vi "Search Or Add Frame.vi"(10 "Detection Frame In 3":T1 {"robots_blue"."height" format="%+4.3f"; "robots_blue"."pixel_y" format="%+4.3f"; "robots_blue"."pixel_x" format="%+4.3f"; "robots_blue"."orientation" format="%+4.3f"; "robots_blue"."y" format="%+4.3f"; "robots_blue"."confidence" format="%4.3f"; "robots_blue"."x" format="%+4.3f"; "robots_yellow"."height" format="%+4.3f"; "robots_yellow"."pixel_y" format="%+4.3f"; "robots_yellow"."pixel_x" format="%+4.3f"; "robots_yellow"."orientation" format="%+4.3f"; "robots_yellow"."y" format="%+4.3f"; "robots_yellow"."confidence" format="%4.3f"; "robots_yellow"."x" format="%+4.3f"}, 11 "Detection Frame In 4":T1[](array[typedef]) {"robots_blue"."height" format="%+4.3f"; "robots_blue"."pixel_y" format="%+4.3f"; "robots_blue"."pixel_x" format="%+4.3f"; "robots_blue"."orientation" format="%+4.3f"; "robots_blue"."y" format="%+4.3f"; "robots_blue"."confidence" format="%4.3f"; "robots_blue"."x" format="%+4.3f"; "robots_yellow"."height" format="%+4.3f"; "robots_yellow"."pixel_y" format="%+4.3f"; "robots_yellow"."pixel_x" format="%+4.3f"; "robots_yellow"."orientation" format="%+4.3f"; "robots_yellow"."y" format="%+4.3f"; "robots_yellow"."confidence" format="%4.3f"; "robots_yellow"."x" format="%+4.3f"}) -> (3 "Detection Frame In 2":T1[](array[typedef]) {"robots_blue"."height" format="%+4.3f"; "robots_blue"."pixel_y" format="%+4.3f"; "robots_blue"."pixel_x" format="%+4.3f"; "robots_blue"."orientation" format="%+4.3f"; "robots_blue"."y" format="%+4.3f"; "robots_blue"."confidence" format="%4.3f"; "robots_blue"."x" format="%+4.3f"; "robots_yellow"."height" format="%+4.3f"; "robots_yellow"."pixel_y" format="%+4.3f"; "robots_yellow"."pixel_x" format="%+4.3f"; "robots_yellow"."orientation" format="%+4.3f"; "robots_yellow"."y" format="%+4.3f"; "robots_yellow"."confidence" format="%4.3f"; "robots_yellow"."x" format="%+4.3f"})   [LabVIEW 2017]
uses:
  SSL Detection Robot.ctl
  SSL Detection Ball.ctl
  SSL Detection Frame.ctl
  <vilib>/Analysis/Matrix/Datatypes/RealMatrix.ctl
  <vilib>/Analysis/Matrix/NI_Matrix.lvlib
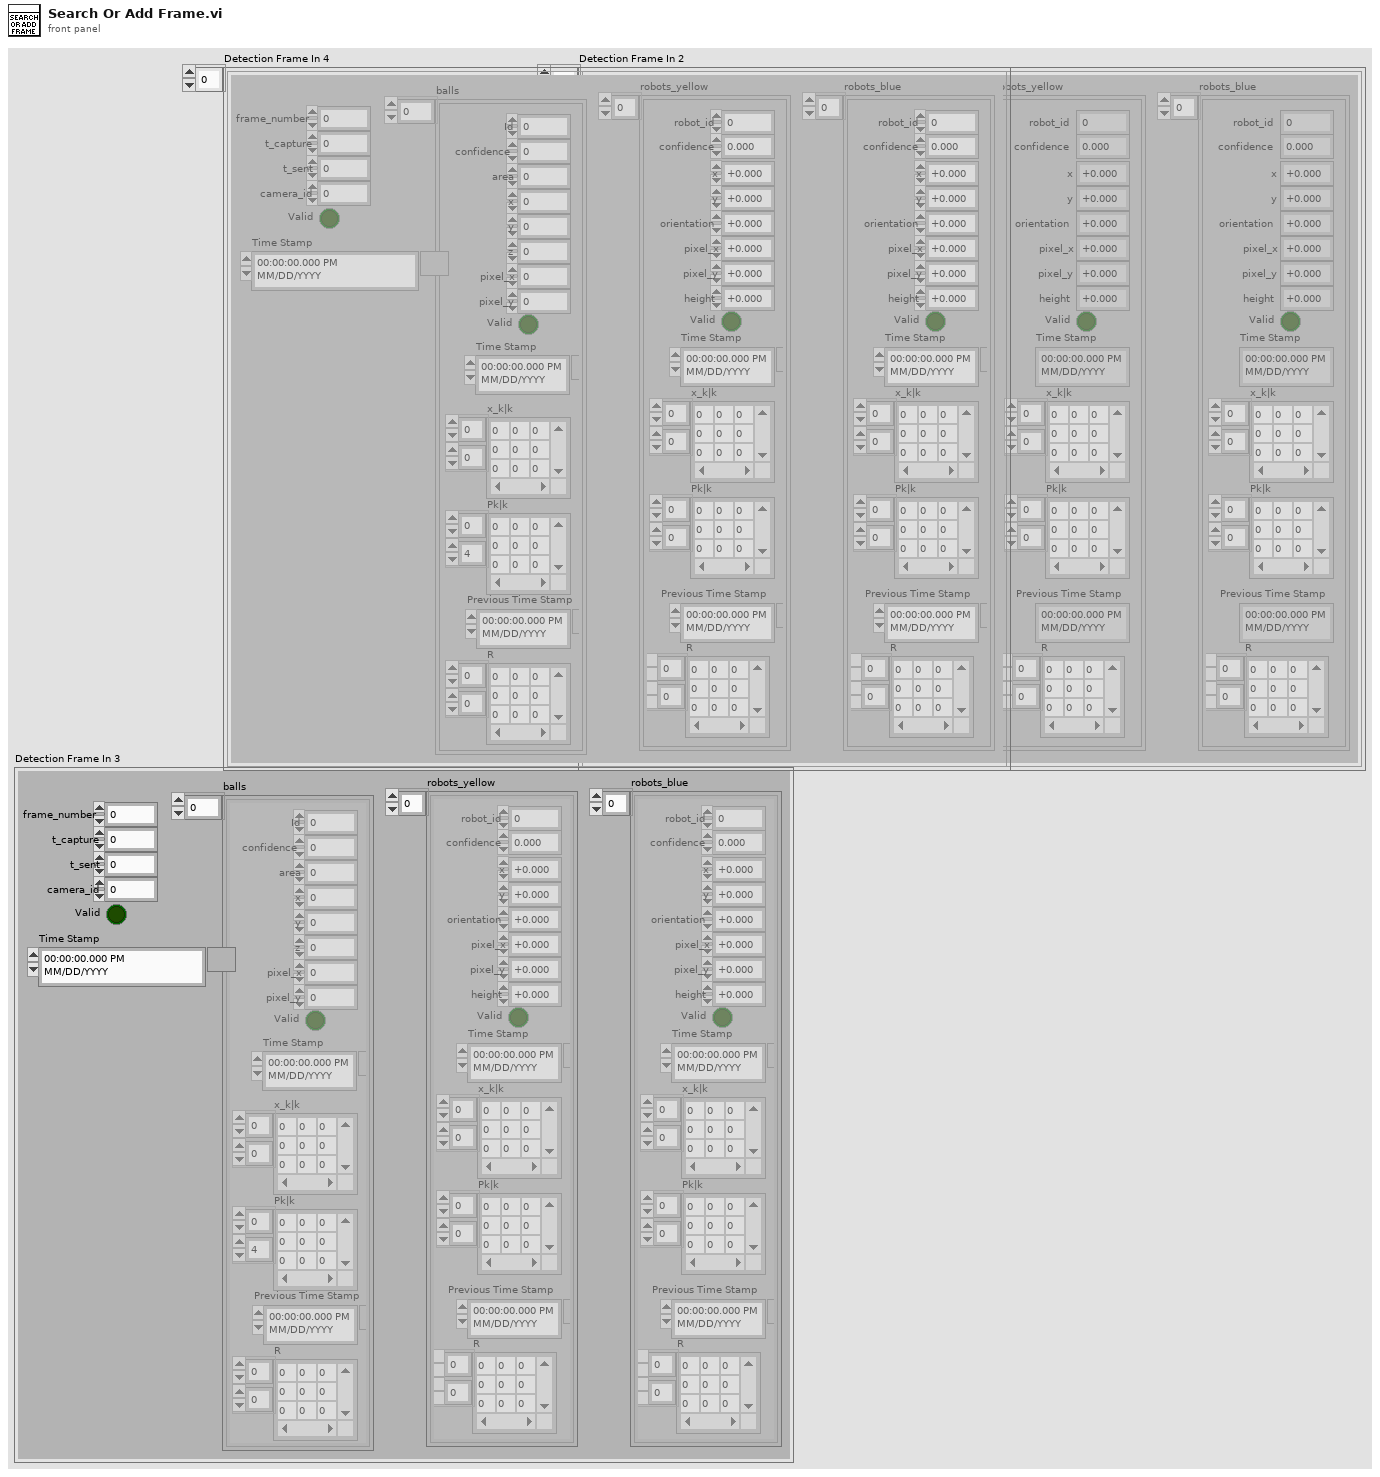
[diagram p1: front panel]
types:
  T1 = typedef "SSL Detection Frame.ctl" = cluster{"frame_number":u32, "t_capture":dbl, "t_sent":dbl, "camera_id":u32, "robots_yellow":T2[], "robots_blue":T2[], "balls":T4[], "Valid":bool, "Time Stamp":timestamp}
  T2 = typedef "SSL Detection Robot.ctl" = cluster{"x":sgl, "robot_id":u32, "confidence":sgl, "y":sgl, "orientation":sgl, "pixel_x":sgl, "pixel_y":sgl, "height":sgl, "Valid":bool, "Time Stamp":timestamp, "x_k|k":T3, "Pk|k":T3, "Previous Time Stamp":timestamp, "R":T3}
  T3 = typedef "NI_Matrix.lvlib/RealMatrix.ctl" = dbl[][]
  T4 = typedef "SSL Detection Ball.ctl" = cluster{"x":sgl, "area":u32, "confidence":sgl, "y":sgl, "z":sgl, "pixel_x":sgl, "pixel_y":sgl, "Valid":bool, "Time Stamp":timestamp, "x_k|k":T3, "Pk|k":T3, "Id":u32, "Previous Time Stamp":timestamp, "R":T3}
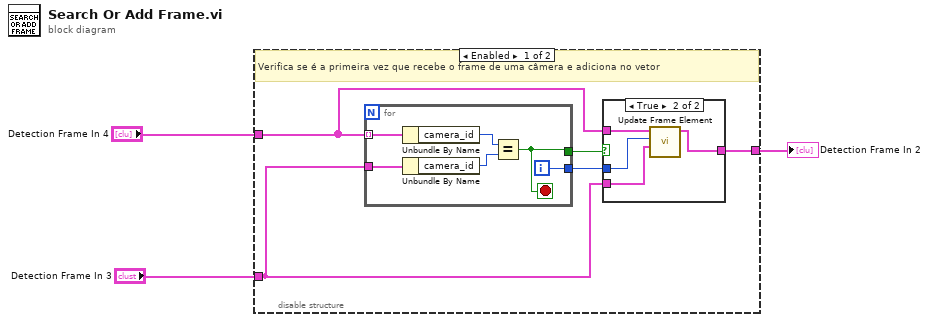
[diagram p0: block diagram]
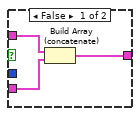
[diagram p2: hidden frame]
diagram:
  n1 = disable-structure "Diagram Disable Structure" shown="Enabled" {
    disable-tunnel: "Detection Frame In 4" -> [w7 _]
    disable-tunnel: "Detection Frame In 3" -> [w5 _]
    disable-tunnel: [w4 _] -> w3
    frame Enabled {
      # "Verifica se é a primeira vez que recebe o frame de uma câmera e adiciona no vetor"
      n2 = for {
        tunnel: w7 -> [w21] mode=indexing
        tunnel: w5 -> [w20]
        tunnel: [w17] -> w8
        tunnel: [w16] -> w6
        i -> [w16]
        stop <- w17 stop-if-true
        n3 = Unbundle By Name(w21) -> ("camera_id"=w19:u32)
        n4 = Unbundle By Name(w20) -> ("camera_id"=w18:u32)
        n5 = Equal?(x=w19, y=w18) -> (x = y?=w17:bool)
      }
      n6 = case shown="True" w8 {
        tunnel: w7 -> [w11 w15]
        tunnel: w5 -> [w9 w13]
        tunnel: [w10 w12] -> w4
        tunnel: w6 -> [_ w14]
        frame False {
          n7 = Build Array (concatenate)(w11, w9) -> (w10:T1[])
        }
        frame True {
          n8 = call "Update Frame Element.vi"("Detection Frame In in"=w13, "Numeric"=w14, "Detection Frame In 3"=w15) -> ("Detection Frame In out"=w12:T1[])  [unwired: 8 in]
        }
      }
    }
    frame Disabled {
    }
  }
  "Detection Frame In 2" <- w3
